vi "Ej_16_Arduino_DAQ_Servo.vi"() -> ()   [LabVIEW 2021]
uses:
  <vilib>/Instr/_visa.llb/VISA Configure Serial Port (Instr).vi
panel:
  out "output 1":dbl
  out "read buffer":string
  out "Waveform Graph 2":dynamicdata(graph)
  in  "Direccion":string[](array[string])
  in  "stop":bool
  out "Waveform Graph":dynamicdata(graph)
  in  "Puerto de la Tarjeta":refnum<visa-resource-name>
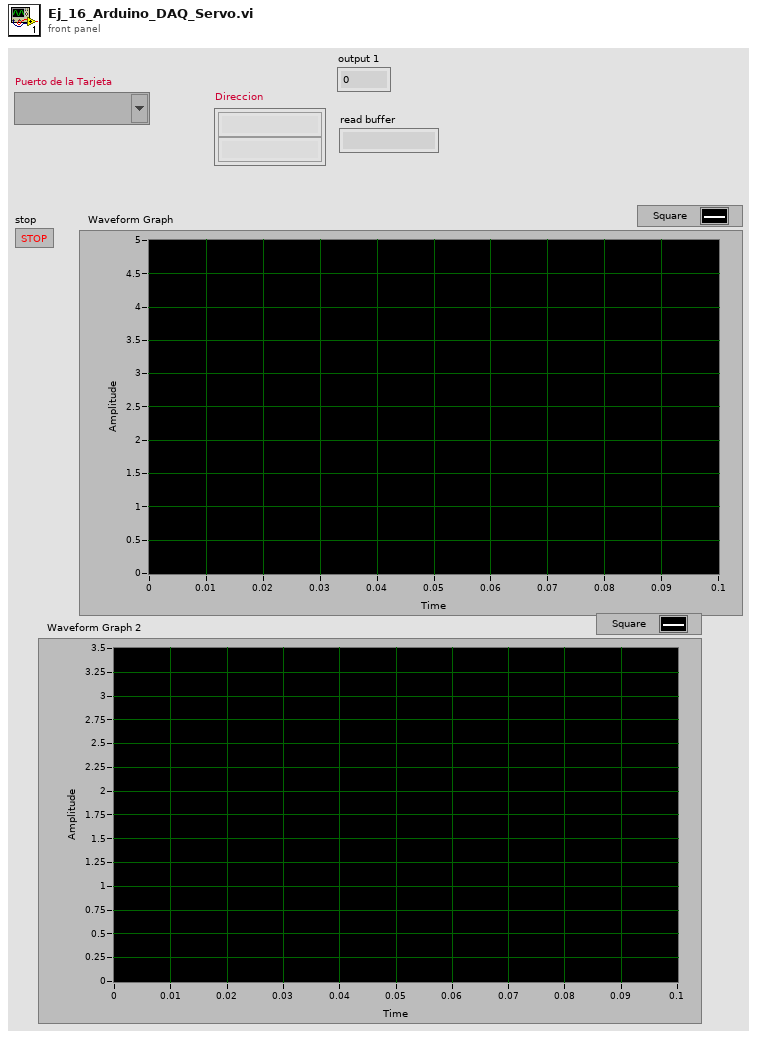
[diagram p1: front panel]
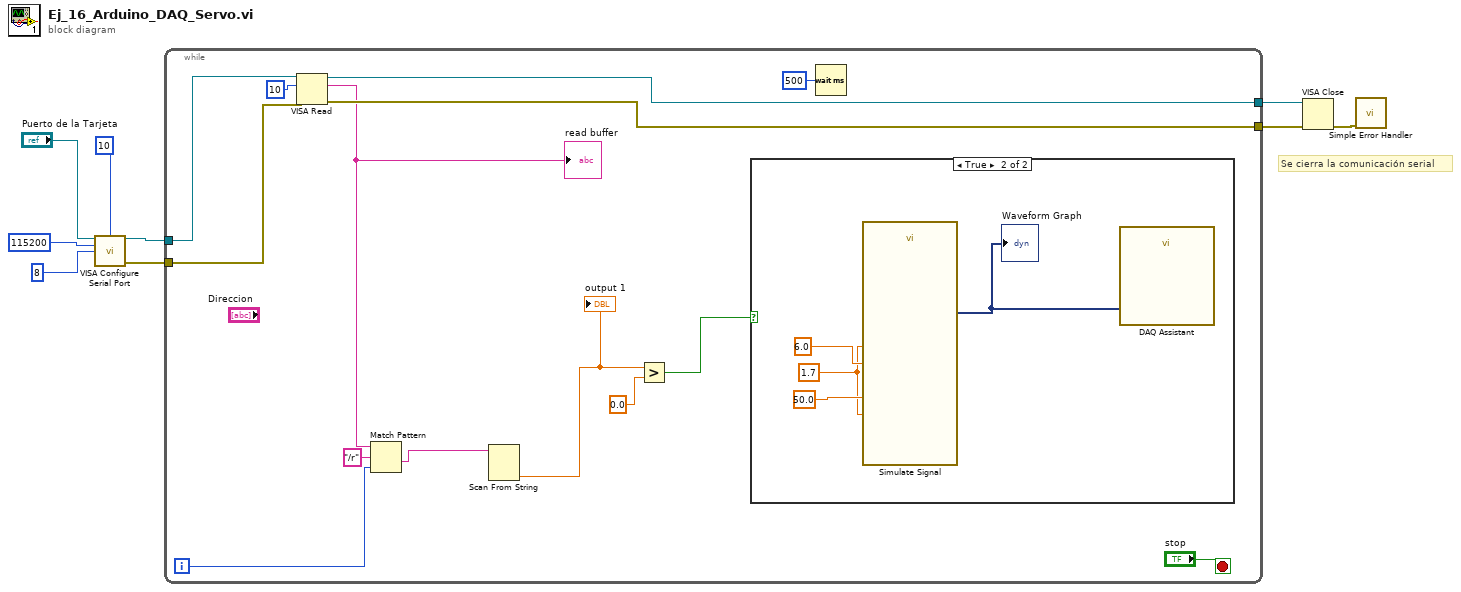
[diagram p0: block diagram]
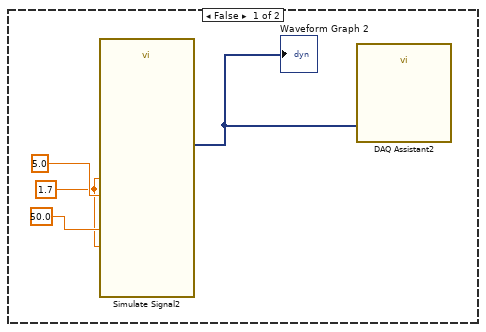
[diagram p2: hidden frame]
diagram:
  # "Se cierra la comunicación serial"
  n1 = call-poly "VISA Configure Serial Port"("VISA resource name"="Puerto de la Tarjeta", "termination char\n(0xA = '\\n' = LF)"=u8 10 ("termination char\n(0xA = '\\n' = LF)"), "baud rate (9600)"=u32 115200, "data bits (8)"=u16 8) -> ("VISA resource name out"=w4:refnum<visa-resource-name>, "error out"=w3:errorcluster)  [unwired: 10 in]
  n2 = while {
    tunnel: w4 -> [w22]
    tunnel: w3 -> [w21]
    tunnel: [w18] -> w2
    tunnel: [w17] -> w1
    i -> [w14]
    stop <- "stop" stop-if-true
    n3 = VISA Read(VISA resource name=w22, byte count=u32 10, error in (no error)=w21) -> (VISA resource name out=w18:refnum<visa-resource-name>, read buffer=w15:string, error out=w17:errorcluster)  [unwired: 1 out]
    "read buffer" <- w15
    n4 = Match Pattern(string=w15, regular expression="/r", offset (0)=w14) -> (after substring=w11:string)  [unwired: 3 out]
    n5 = Scan From String(input string=w11) -> (output 1=w13:dbl)  [unwired: 4 in, 3 out]
    "output 1" <- w13
    n6 = Greater?(x=w13, y=0.0) -> (0:w19:bool)
    n7 = case shown="True" w19 {
      frame False {
        w24 = 1.7 ("Amplitud")
        n8 = call "Simulate Signal2"("Offset"=w24, "Duty Cycle (%)"=5.0, "Frequency"=50.0, "Amplitude"=w24) -> ("Square"=w25:dynamicdata)  [unwired: 10 in, 1 out]
        "Waveform Graph 2" <- w25
        n9 = call "DAQ Assistant2"("data"=w25) -> ()  [unwired: 17 in, 2 out]
      }
      frame True {
        w28 = 1.7 ("Amplitud")
        n10 = call "Simulate Signal"("Offset"=w28, "Duty Cycle (%)"=6.0, "Frequency"=50.0, "Amplitude"=w28) -> ("Square"=w29:dynamicdata)  [unwired: 10 in, 1 out]
        "Waveform Graph" <- w29
        n11 = call "DAQ Assistant"("data"=w29) -> ()  [unwired: 17 in, 2 out]
      }
    }
    n12 = Wait (ms)(milliseconds to wait=u32 500) -> ()  [unwired: 1 out]
  }
  n13 = VISA Close(VISA resource name=w2, error in (no error)=w1) -> (error out=w5:errorcluster)
  n14 = call <vilib>:"Simple Error Handler.vi"("error in (no error)"=w5) -> ()  [unwired: 4 in, 5 out]
